vi "Beta 3.1.vi"() -> ()   [LabVIEW 2011]
uses:
  <vilib>/vision/NI_Vision_Development_Module.lvlib
panel:
  out "XY Graph 2":cluster{dbl[], dbl[]}(graph)
  in  "Structuring Element":dbl[][](array[numeric])=[[0.0, 1.0, 0.0], [1.0, 1.0, 1.0], [0.0, 1.0, 0.0]]
  in  "Morphology":u16(ring) items=["(none)", "AutoM", "Close", "Dilate", "Erode", "Gradient", "Gradient out", "Gradient in", "Open", "Thick", "Thin"]
  in  "Generate":bool
  in  "Look for":enum16{"Bright Objects", "Dark Objects"}(ring)
  in  "Method":T1(ring)=enum."Inter-class Variance"
  out "Binary":T2(plugin-control)
  in  "Stop":bool
  in  "Browse":bool
  out "Original Image":T2(plugin-control)
  out "Path to Image":path
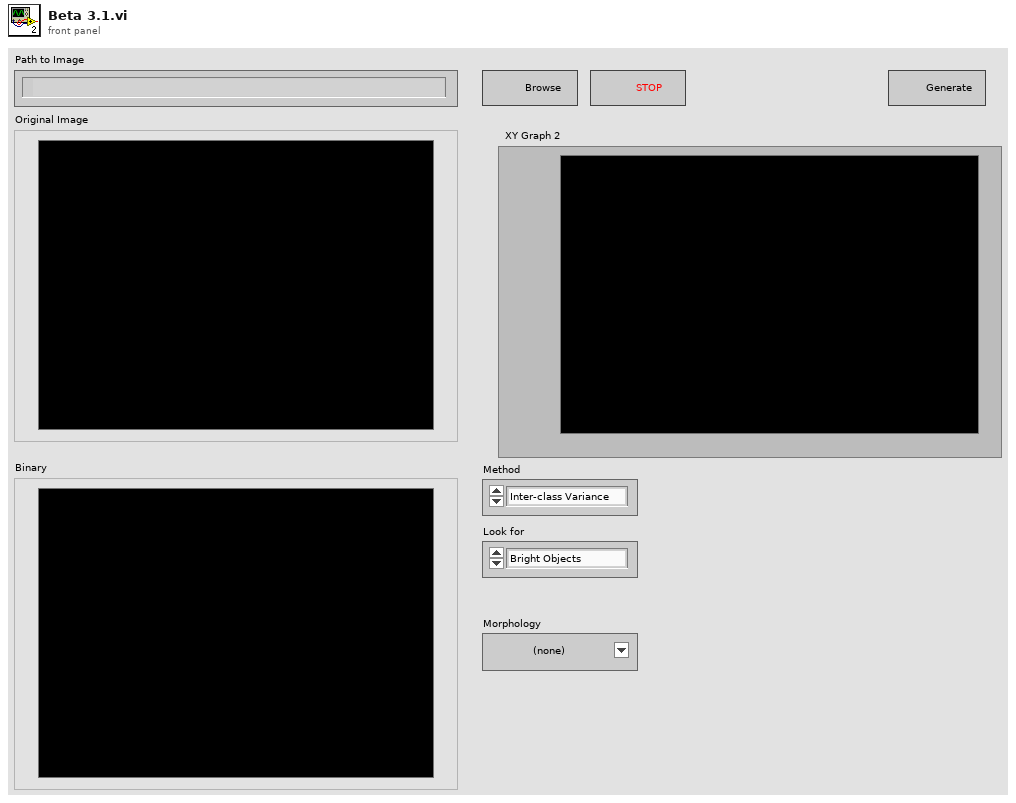
[diagram p1: front panel]
types:
  T1 = enum16{"Clustering", "Entropy", "Metric", "Moments", "Inter-class Variance"}
  T2 = typedef "IMAQ Image.ctl" = refnum<image>
  T3 = typedef "Image Type" = u32
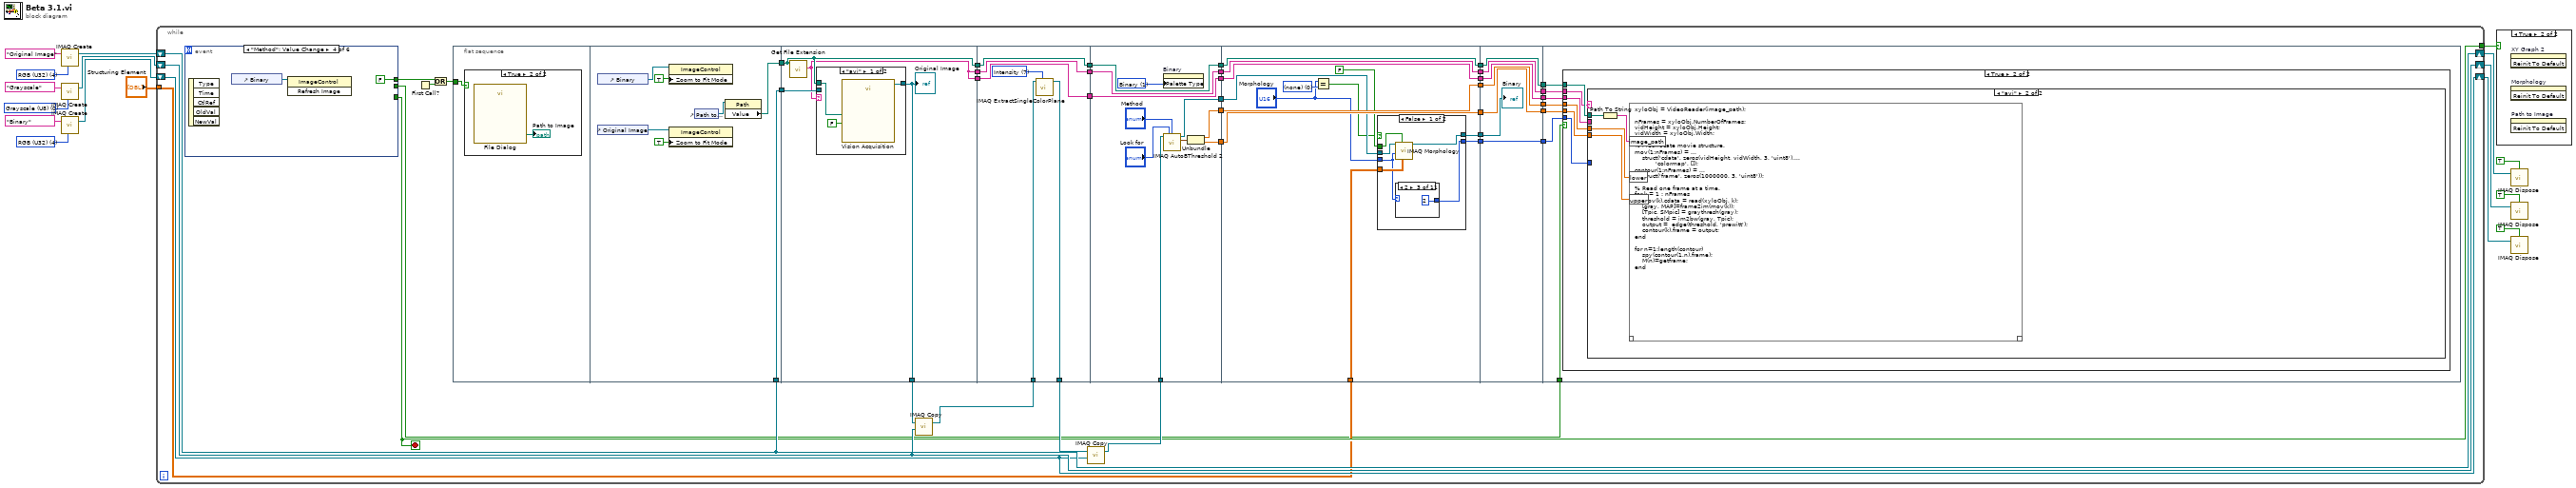
[diagram p0: block diagram]
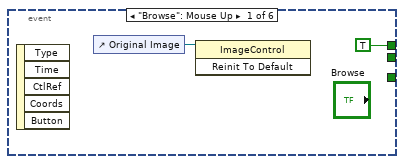
[diagram p3: hidden frame]
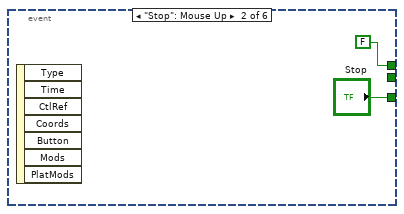
[diagram p4: hidden frame]
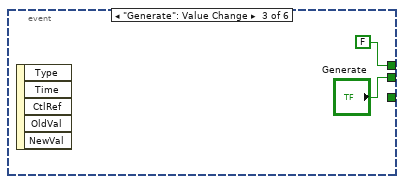
[diagram p5: hidden frame]
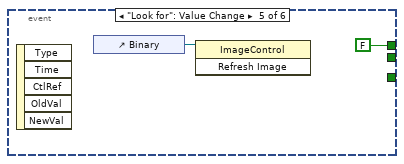
[diagram p6: hidden frame]
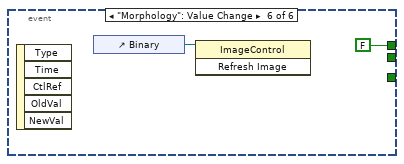
[diagram p7: hidden frame]
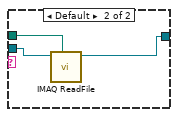
[diagram p9: hidden frame]
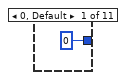
[diagram p10: hidden frame]
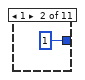
[diagram p11: hidden frame]
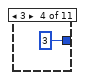
[diagram p12: hidden frame]
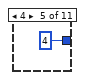
[diagram p13: hidden frame]
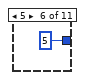
[diagram p14: hidden frame]
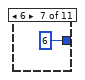
[diagram p15: hidden frame]
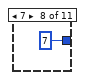
[diagram p16: hidden frame]
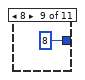
[diagram p17: hidden frame]
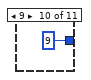
[diagram p18: hidden frame]
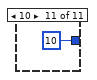
[diagram p19: hidden frame]
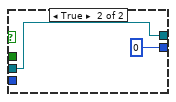
[diagram p20: hidden frame]
diagram:
  w5 = T3 4 items=["Grayscale (U8)", "Grayscale (I16)", "Grayscale (SGL)", "Complex (CSG)", "RGB (U32)", "HSL (U32)", "RGB (U64)", "Grayscale (U16)"] ("Image Type")
  w11 = T3 0 items=["Grayscale (U8)", "Grayscale (I16)", "Grayscale (SGL)", "Complex (CSG)", "RGB (U32)", "HSL (U32)", "RGB (U64)", "Grayscale (U16)"] ("Image Type")
  w16 = T3 4 items=["Grayscale (U8)", "Grayscale (I16)", "Grayscale (SGL)", "Complex (CSG)", "RGB (U32)", "HSL (U32)", "RGB (U64)", "Grayscale (U16)"] ("Image Type")
  n1 = call "IMAQ Create"("Image Name"="Original Image", "Image Type"=w16) -> ("New Image"=w15:T2)  [unwired: 3 in, 1 out]
  n2 = call "IMAQ Create"("Image Name"="Grayscale", "Image Type"=w11) -> ("New Image"=w10:T2)  [unwired: 3 in, 1 out]
  n3 = call "IMAQ Create"("Image Name"="Binary", "Image Type"=w5) -> ("New Image"=w2:T2)  [unwired: 3 in, 1 out]
  n4 = while {
    shift-right: [w52] -> w14
    shift-left: w15 -> [w52]
    tunnel: [w33] -> w13
    shift-right: [w47] -> w8
    shift-left: w10 -> [w47]
    shift-right: [w42] -> w3
    shift-left: w2 -> [w42]
    tunnel: "Structuring Element" -> [w32]
    stop <- w33 stop-if-true
    n5 = event shown="[3] \"Method\": Value Change" {
      selector: _ -> [_ _ _ _ _ _]
      dyn-events: _ -> [_ _ _ _ _ _]
      timeout: _ -> [_ _ _ _ _ _]
      tunnel: [TRUE FALSE FALSE FALSE FALSE FALSE] -> w56
      tunnel: [_ "Stop" _ _ _ _] -> w33
      tunnel: [_ _ "Generate" _ _ _] -> w18
      event "Browse": Mouse Up {
        n6 = event-data() -> ()  [unwired: 1 in, 5 out]
        n7 = control-ref of="Original Image"() -> (w59:refnum<vi>)
        n8 = invoke class="ImageControl" method="Reinit To Default"(reference=w59) -> ()  [unwired: 2 in, 3 out]
      }
      event "Stop": Mouse Up {
        n9 = event-data() -> ()  [unwired: 1 in, 7 out]
      }
      event "Generate": Value Change {
        n10 = event-data() -> ()  [unwired: 1 in, 5 out]
      }
      event "Method": Value Change {
        n11 = event-data() -> ()  [unwired: 1 in, 5 out]
        n12 = control-ref of="Binary"() -> (w64:refnum<vi>)
        n13 = invoke class="ImageControl" method="Refresh Image"(reference=w64) -> ()  [unwired: 2 in, 3 out]
      }
      event "Look for": Value Change {
        n14 = event-data() -> ()  [unwired: 1 in, 5 out]
        n15 = control-ref of="Binary"() -> (w66:refnum<vi>)
        n16 = invoke class="ImageControl" method="Refresh Image"(reference=w66) -> ()  [unwired: 2 in, 3 out]
      }
      event "Morphology": Value Change {
        n17 = event-data() -> ()  [unwired: 1 in, 5 out]
        n18 = control-ref of="Binary"() -> (w68:refnum<vi>)
        n19 = invoke class="ImageControl" method="Refresh Image"(reference=w68) -> ()  [unwired: 2 in, 3 out]
      }
    }
    n20 = First Call?() -> (First Call?: T/F=w55:bool)
    n21 = Or(x=w56, y=w55) -> (x .or. y?=w54:bool)
    n22 = flat-sequence {
      tunnel: w54 -> [w70]
      tunnel: [w74] -> w57
      tunnel: [w75] -> w53
      tunnel: w52 -> [w74]
      tunnel: w57 -> [w82]
      tunnel: w53 -> [w81]
      tunnel: [w81] -> w51
      tunnel: [w80] -> w29
      tunnel: [w79] -> w24
      tunnel: [w79] -> w19
      tunnel: w51 -> [w94]
      tunnel: [w94] -> w50
      tunnel: w48 -> [w92]
      tunnel: [w91] -> w43
      tunnel: [w90] -> w25
      tunnel: w24 -> [w90]
      tunnel: [w89] -> w20
      tunnel: w19 -> [w89]
      tunnel: w50 -> [w105]
      tunnel: [w105] -> w41
      tunnel: [w104] -> w39
      tunnel: [w99] -> w38
      tunnel: [w98] -> w36
      tunnel: w44 -> [w97]
      tunnel: [w96] -> w26
      tunnel: w25 -> [w96]
      tunnel: [w95] -> w21
      tunnel: w20 -> [w95]
      tunnel: w41 -> [w118]
      tunnel: [w118] -> w40
      tunnel: w39 -> [w115]
      tunnel: w38 -> [w117]
      tunnel: [w117] -> w37
      tunnel: w36 -> [w116]
      tunnel: [w116] -> w35
      tunnel: [w114] -> w34
      tunnel: w32 -> [w109]
      tunnel: [w108] -> w31
      tunnel: [w107] -> w27
      tunnel: w26 -> [w107]
      tunnel: [w106] -> w22
      tunnel: w21 -> [w106]
      tunnel: w40 -> [w144]
      tunnel: [w144] -> w49
      tunnel: [w143] -> w46
      tunnel: w37 -> [w143]
      tunnel: [w142] -> w45
      tunnel: w35 -> [w142]
      tunnel: w34 -> [w141]
      tunnel: w31 -> [w140]
      tunnel: [w140] -> w30
      tunnel: [w139] -> w28
      tunnel: w27 -> [w139]
      tunnel: [w138] -> w23
      tunnel: w22 -> [w138]
      tunnel: w49 -> [w151]
      tunnel: w46 -> [w150]
      tunnel: w45 -> [w149]
      tunnel: w30 -> [w148]
      tunnel: w28 -> [w147]
      tunnel: w23 -> [w146]
      tunnel: w18 -> [w145]
      frame #0 {
        n23 = case shown="True" w70 {
          frame False {
          }
          frame True {
            n24 = call "File Dialog"() -> ("selected path"=→"Path to Image":path)  [unwired: 12 in, 3 out]
          }
        }
      }
      frame #1 {
        n25 = control-ref of="Binary"() -> (w73:refnum<vi>)
        n26 = control-ref of="Original Image"() -> (w78:refnum<vi>)
        n27 = property class="ImageControl"(reference=w73, "Zoom to Fit Mode"=TRUE) -> ()  [unwired: 1 in, 2 out]
        n28 = property class="ImageControl"(reference=w78, "Zoom to Fit Mode"=TRUE) -> ()  [unwired: 1 in, 2 out]
        n29 = control-ref of="Path to Image"() -> (w76:refnum<vi>)
        n30 = property class="Path"(reference=w76) -> ("Value"=w75:path)  [unwired: 1 in, 2 out]
      }
      frame #2 {
        n31 = call <vilib>:"Get File Extension.vi"("file"=w81) -> ("lowercase file extension"=w79:string)  [unwired: 7 in, 3 out]
        n32 = case shown="\"avi\"" w79 {
          tunnel: w82 -> [_ w88]
          tunnel: w81 -> [w85 w87]
          tunnel: [w84 w86] -> w80
          frame "avi" {
            n33 = call "Vision Acquisition"("AVI Path"=w85, "Stop (F)"=FALSE) -> ("Image Out"=w84:T2)  [unwired: 1 in, 24 out]
          }
          frame Default {
            n34 = call "IMAQ ReadFile"("File Path"=w87, "Image"=w88) -> ("Image Out"=w86:T2)  [unwired: 5 in, 4 out]
          }
        }
        "Original Image" <- w80
      }
      frame #3 {
        w93 = 7 items=["Red", "Green", "Blue", "Hue", "Saturation", "Luminance", "Value", "Intensity"] ("Color Plane")
        n35 = call "IMAQ ExtractSingleColorPlane"("Color Plane"=w93, "Image Src"=w92) -> ("Image Dst Out"=w91:T2)  [unwired: 8 in, 1 out]
      }
      frame #4 {
        w103 = u32 1 items=["Grayscale", "Binary", "Gradient", "Rainbow", "Temperature", "User Defined"] ("Palette")
        n36 = property on="Binary" class="ImageControl"("Palette Type"=w103) -> ()  [unwired: 2 in, 2 out]
        n37 = call "IMAQ AutoBThreshold 2"("Image Src"=w97, "Look For (Bright Objects)"="Look for", "Method (clustering)"="Method") -> ("Image Dst Out"=w104:T2, "Threshold Range Out"=w100:cluster{"Lower value":sgl, "Upper value":sgl})  [unwired: 10 in, 1 out]
        n38 = Unbundle(w100) -> ("Lower value"=w99:sgl, "Upper value"=w98:sgl)
      }
      frame #5 {
        w112 = u16 0 items=["(none)"]
        n39 = Equal?(x="Morphology", y=w112) -> (x = y?=w111:bool)
        n40 = case shown="False" w111 {
          tunnel: w115 -> [w122 w137]
          tunnel: [w123 w137] -> w114
          tunnel: FALSE -> [w124 _]
          tunnel: "Morphology" -> [w120 _]
          tunnel: w109 -> [w121 _]
          tunnel: [w119 0] -> w108
          frame False {
            n41 = call "IMAQ Morphology"("Structuring Element"=w121, "Square/Hexa (Square)"=w124, "Operation"=w120, "Image Src"=w122) -> ("Image Dst Out"=w123:T2)  [unwired: 6 in, 1 out]
            n42 = case shown="2" w120 {
              tunnel: [0 1 2 3 4 5 6 7 8 9 10] -> w119
              frame 0, Default {
              }
              frame 1 {
              }
              frame 2 {
              }
              frame 3 {
              }
              frame 4 {
              }
              frame 5 {
              }
              frame 6 {
              }
              frame 7 {
              }
              frame 8 {
              }
              frame 9 {
              }
              frame 10 {
              }
            }
          }
          frame True {
          }
        }
      }
      frame #6 {
        "Binary" <- w141
      }
      frame #7 {
        n43 = case shown="True" w145 {
          tunnel: w151 -> [_ w157]
          tunnel: w150 -> [_ w156]
          tunnel: w149 -> [_ w155]
          tunnel: w148 -> [_ w154]
          tunnel: w147 -> [_ w153]
          tunnel: w146 -> [_ w152]
          frame False {
          }
          frame True {
            n44 = case shown="\"avi\"" w152 {
              tunnel: w157 -> [w174 w178]
              tunnel: w156 -> [w173 w177]
              tunnel: w155 -> [w172 w176]
              tunnel: w154 -> [w171 _]
              tunnel: w153 -> [w170 _]
              frame Default {
                n45 = Path To String(path=w174) -> (string=w169:string)
                n46 = Reverse String(1:w169) -> (0:w168:string)
                n47 = Search/Split String(string=w168, search string/char (-)="\\") -> (substring before match=w166:string, match + rest of string=w165:string)  [unwired: 1 in, 1 out]
                n48 = Reverse String(1:w166) -> (0:w164:string)
                n49 = Reverse String(1:w165) -> (0:w163:string)
                n50 = script code="original = imread(strcat(image_path, '\\', image_name));\ngray = rgb2gray(original);\n\ngray_adjusted = imadjust(gray);\nthreshold = (gray_adjusted>=lower & gray_adjusted<=upper);\nse = strel('disk', 1);\nswitch morph_n\ncase 0\nmorphed = threshold;\ncase 1\nmorphed = threshold;\ncase 2\nmorphed = imclose(threshold, se);\ncase 3\nmorphed = imdilate(threshold, se);\ncase 4\nmorphed = imerode(threshold, se);\ncase 5\nmorphed = imdilate(threshold, se) - imerode(threshold, se);\ncase 6\nmorphed = imdilate(threshold, se) - threshold;\ncase 7\nmorphed = threshold - imerode(threshold, se);\ncase 8\nmorphed = imopen(threshold, se);\ncase 9\nmorphed = bwmorph(threshold, 'thicken', 1);\ncase 10\nmorphed = bwmorph(threshold, 'thin', 1);\notherwise\nmorphed = threshold;\nend\n\nflip = flipud(morphed);\ncontour = edge(flip, 'prewitt');\n[i, j] = ind2sub(size(contour), find(contour==1));\ncoordinate =  [j, i];"("image_name"=w164, "image_path"=w163, "lower"=w173, "upper"=w172, "morph_n"=w171, "file_type"=w170) -> ("coordinate"=w162:dbl[][])  [unwired: 1 in, 1 out]
                n51 = Index Array(array=w162, index (col) #1=0 ("disabled index (col)")) -> (element #1=w161:dbl[], element #2=w160:dbl[])  [unwired: 3 in]
                n52 = Bundle(w161, w160) -> (→"XY Graph 2":cluster{dbl[], dbl[]})  [unwired: 1 in]
              }
              frame "avi" {
                n53 = Path To String(path=w178) -> (string=w175:string)
                n54 = script code="xyloObj = VideoReader(image_path);\n\nnFrames = xyloObj.NumberOfFrames;\nvidHeight = xyloObj.Height;\nvidWidth = xyloObj.Width;\n\n% Preallocate movie structure.\nmov(1:nFrames) = ...\n    struct('cdata', zeros(vidHeight, vidWidth, 3, 'uint8'),...\n           'colormap', []);\ncontour(1:nFrames) = ...\n    struct('frame', zeros(1000000, 3, 'uint8'));\n\n% Read one frame at a time.\nfor k = 1 : nFrames\n    mov(k).cdata = read(xyloObj, k);\n    [gray, MAP]=frame2im(mov(k));\n    [Tpic, SMpic] = graythresh(gray);\n    threshold = im2bw(gray, Tpic);\n    output =  edge(threshold, 'prewitt');\n    contour(k).frame = output;\nend\n\nfor n=1:length(contour)\n    spy(contour(1,n).frame);\n    M(n)=getframe;\nend"("image_path"=w175, "lower"=w177, "upper"=w176) -> ()  [unwired: 1 in, 1 out]
              }
            }
          }
        }
      }
    }
    n55 = call "IMAQ Copy"("Image Dst"=w47, "Image Src"=w29) -> ("Image Dst Out"=w48:T2)  [unwired: 4 in, 1 out]
    n56 = call "IMAQ Copy"("Image Dst"=w42, "Image Src"=w43) -> ("Image Dst Out"=w44:T2)  [unwired: 4 in, 1 out]
  }
  n57 = case shown="True" w13 {
    frame False {
    }
    frame True {
      n58 = invoke on="XY Graph 2" class="XYGraph (strict)" method="Reinit To Default"() -> ()  [unwired: 3 in, 3 out]
      n59 = invoke on="Morphology" class="Ring (strict)" method="Reinit To Default"() -> ()  [unwired: 3 in, 3 out]
      n60 = invoke on="Path to Image" class="Path" method="Reinit To Default"() -> ()  [unwired: 3 in, 3 out]
    }
  }
  n61 = call "IMAQ Dispose"("All Images? (No)"=TRUE, "Image"=w14) -> ()  [unwired: 4 in, 1 out]
  n62 = call "IMAQ Dispose"("All Images? (No)"=TRUE, "Image"=w8) -> ()  [unwired: 4 in, 1 out]
  n63 = call "IMAQ Dispose"("All Images? (No)"=TRUE, "Image"=w3) -> ()  [unwired: 4 in, 1 out]
